vi "Cam_Size.vi"(8 "error in (no error)":errorcluster, 11 "Image Size":T1(ring)) -> (0 "error out":errorcluster, 2 "h":i32=320, 3 "w":i32=480)   [LabVIEW 2014, in "QwaveSys RPi Training Library.lvlib"]
uses:
  <vilib>/Q-Wave Systems/QwaveSys RPi Training Package (Demo)/Addons/QwaveSys RPi Training Library.lvlib
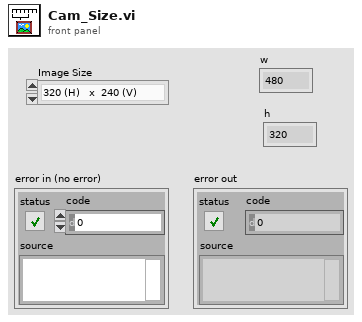
[diagram p1: front panel]
types:
  T1 = enum16{"320 (H)   x  240 (V)", "352(H)    x  288 (V)", "640 (H)   x  480 (V) ", "800 (H)   x  600 (V)", "1024 (H) x  768 (V)", "1280 (H) x  720 (V)", "1280 (H) x 1024 (V)", "1920 (H) x 1080 (V)"}
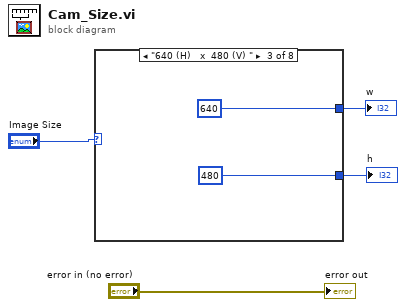
[diagram p0: block diagram]
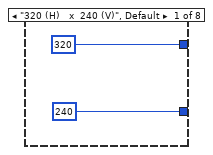
[diagram p2: hidden frame]
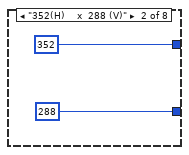
[diagram p3: hidden frame]
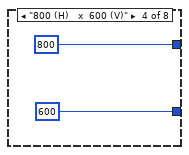
[diagram p4: hidden frame]
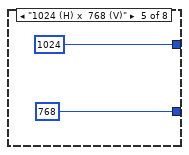
[diagram p5: hidden frame]
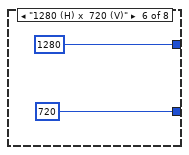
[diagram p6: hidden frame]
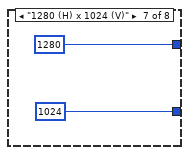
[diagram p7: hidden frame]
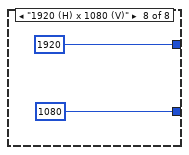
[diagram p8: hidden frame]
diagram:
  n1 = case shown="\"640 (H)   x  480 (V) \"" "Image Size" {
    tunnel: [320 352 640 800 1024 1280 1280 1920] -> w3
    tunnel: [240 288 480 600 768 720 1024 1080] -> w2
    frame "320 (H)   x  240 (V)", Default {
    }
    frame "352(H)    x  288 (V)" {
    }
    frame "640 (H)   x  480 (V) " {
    }
    frame "800 (H)   x  600 (V)" {
    }
    frame "1024 (H) x  768 (V)" {
    }
    frame "1280 (H) x  720 (V)" {
    }
    frame "1280 (H) x 1024 (V)" {
    }
    frame "1920 (H) x 1080 (V)" {
    }
  }
  "w" <- w3
  "h" <- w2
  "error out" <- "error in (no error)"
